vi "Actor Receive Core.vi"(10 "Msg in":refnum<class "Msg Strategy.lvclass">, 11 "Self Actor State in":refnum<class "Self Actor State.lvclass">) -> (2 "Msg out":refnum<class "Msg Strategy.lvclass">)   [LabVIEW 2021, in "jettl.lvlib" / "Self Actor State.lvclass"]
uses:
  Self Actor State.lvclass
  Msg Strategy/Msg Strategy.lvclass
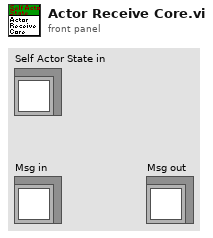
[diagram p1: front panel]
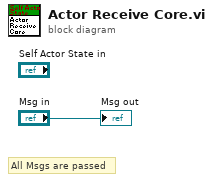
[diagram p0: block diagram]
diagram:
  # "All Msgs are passed"
  "Msg out" <- "Msg in"
